vi "two stepper.vi"() -> ()   [LabVIEW 2018]
uses:
  <vilib>/LabVIEW Interface for Arduino/Type Defs/Board Type.ctl
  <vilib>/LabVIEW Interface for Arduino/Type Defs/Connection Type.ctl
  <vilib>/LabVIEW Interface for Arduino/LabVIEW Interface for Arduino.lvlib
panel:
  out "# steps moved":i32
  in  "OK Button":bool
  in  "?":i8(slide) step=2 scale=0.0..2.0
  in  "MOTION":bool
  out "stop motion":bool
  out "Moving?":bool
  in  "Stop":bool
  in  "Arbitray Movement":bool
  in  "# of Steps to Move":i16
  out "Error":errorcluster
  in  "# of translation Steps":i16
  out "Steps Remaining?":bool
  out "Iteration #":i32
  in  "Baud Rate":u32=115200
  out "Step Angle":dbl
  in  "Step Size":i16
  out "Steps Remaining?":bool
  in  "Set Speed (Steps/s)":i16=100 min=0 max=3000 step=50
  in  "Steps for 1 rotation":i16
  in  "Board Type (Uno)":T1
  in  "VISA resource":refnum<visa-resource-name>
  # "For Rotational motion"
  # "For Translational Motion"
  # "OFF"
  # "ON"
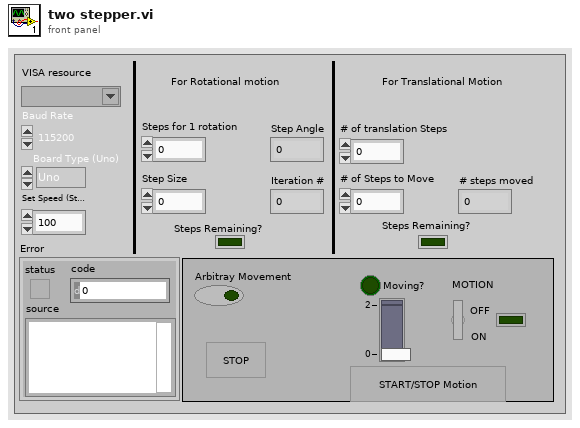
[diagram p1: front panel]
types:
  T1 = typedef "LabVIEW Interface for Arduino.lvlib/Board Type.ctl" = enum16{"Uno", "Dimuelanove w/Atmega 328", "Mega 2560"}
  T2 = typedef "LabVIEW Interface for Arduino.lvlib/Connection Type.ctl" = enum8{"USB / Serial", "XBEE", "BlueSmirf (Bluetooth)"}
  T3 = typedef "LabVIEW Interface for Arduino.lvlib/Arduino Resource.ctl" = cluster{"VISA resource":refnum<visa-resource-name>, "Board Type":T1, "Connection Type":enum8{"USB / Serial"}, "Bytes Per Packet (15)":u8}
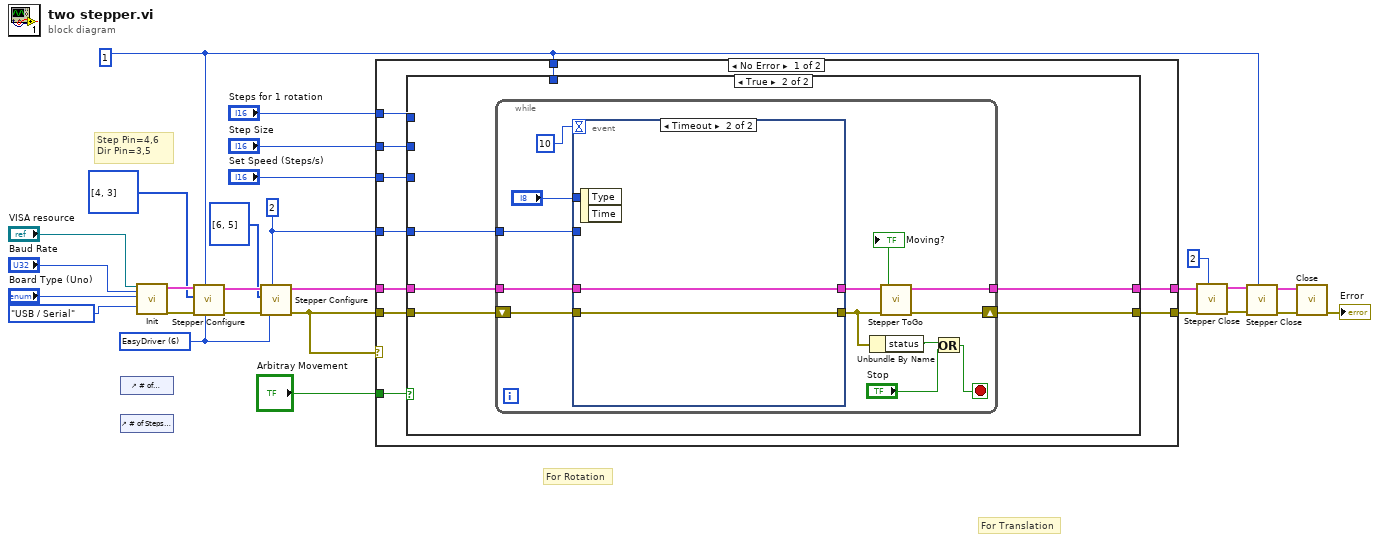
[diagram p0: block diagram]
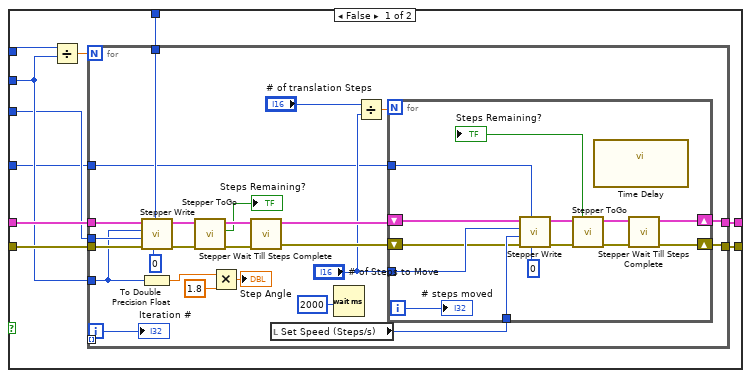
[diagram p2: hidden frame]
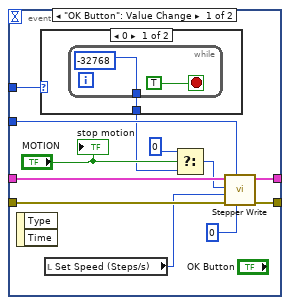
[diagram p3: hidden frame]
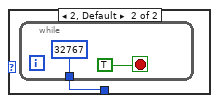
[diagram p4: hidden frame]
diagram:
  w1 = u8 2 ("Stepper #")
  w4 = u8 1 ("Stepper #")
  w2 = u8 6 items=["2 Wire (Pulse & Direction)"=1, "2 Wire"=2, "4 Wire"=4, "EasyDriver"=6, "AF Motor Shield (Stepper 1 & 2 Only)"=5] ("Control Method")
  # "For Translation"
  # "For Rotation"
  # "Step Pin=4,6\nDir Pin=3,5"
  n1 = control-ref of="# of translation Steps"() -> ()  [unwired: 1 out]
  n2 = control-ref of="# of Steps to Move"() -> ()  [unwired: 1 out]
  n3 = call <vilib>:"Init.vi"("VISA resource"="VISA resource", "Baud Rate (115200)"="Baud Rate", "Board Type (Uno)"="Board Type (Uno)", "Connection Type (USB/Serial)"=Connection_Type."USB / Serial") -> ("Arduino Resource"=w24:T3, "error out"=w23:errorcluster)  [unwired: 14 in]
  n4 = call <vilib>:"Stepper Configure.vi"("Control Method"=w2, "Stepper #"=w4, "error in"=w23, "Stepper Pins"=u8[] [4, 3], "Arduino Resource"=w24) -> ("error out"=w6:errorcluster, "Arduino Resource Out"=w8:T3)  [unwired: 5 in]
  n5 = call <vilib>:"Stepper Configure.vi"("Control Method"=w2, "Stepper #"=w1, "error in"=w6, "Stepper Pins"=u8[] [6, 5], "Arduino Resource"=w8) -> ("error out"=w5:errorcluster, "Arduino Resource Out"=w7:T3)  [unwired: 5 in]
  n6 = case shown="No Error" w5 {
    tunnel: [w29 w126] -> w15
    tunnel: [w37 w125] -> w14
    tunnel: w5 -> [w36 w126]
    tunnel: w7 -> [w35 w125]
    tunnel: "Step Size" -> [w34 _]
    tunnel: "Steps for 1 rotation" -> [w33 _]
    tunnel: "Set Speed (Steps/s)" -> [w32 _]
    tunnel: "Arbitray Movement" -> [w31 _]
    tunnel: w4 -> [w30 _]
    tunnel: w1 -> [w28 _]
    frame No Error {
      n7 = case shown="True" w31 {
        tunnel: [w46 w91] -> w37
        tunnel: w36 -> [w45 w88]
        tunnel: w35 -> [w44 w89]
        tunnel: w34 -> [w42 _]
        tunnel: w33 -> [w41 _]
        tunnel: w32 -> [w40 _]
        tunnel: w30 -> [w39 _]
        tunnel: [w47 w90] -> w29
        tunnel: w28 -> [w38 w87]
        frame False {
          n8 = Divide(x=w41, y=w42) -> (x/y=w43:dbl)
          n9 = for {
            N: w43 -> [_]
            tunnel: [w57] -> w47
            tunnel: [w58] -> w46
            tunnel: w45 -> [w69]
            tunnel: w40 -> [w68]
            tunnel: w44 -> [w67]
            tunnel: [w61] -> _ mode=indexing
            tunnel: w42 -> [w60]
            tunnel: w39 -> [w50]
            tunnel: w38 -> [w49]
            i -> [w61]
            n10 = call <vilib>:"Stepper Write.vi"("Set Acceleration (0 to disable)"=i16 0 ("Acceleration"), "Stepper #"=w50, "error in"=w69, "Set Speed (Steps per Second)"=w68, "# of Steps to Move"=w60, "Arduino Resource"=w67) -> ("error out"=w66:errorcluster, "Arduino Resource Out"=w65:T3)  [unwired: 4 in]
            n11 = To Double Precision Float(number=w60) -> (double precision float=w63:dbl)
            n12 = call <vilib>:"Stepper ToGo.vi"("error in"=w66, "Arduino Resource"=w65) -> ("error out"=w72:errorcluster, "Steps Remaining?"=→"Steps Remaining?":bool, "Arduino Resource Out"=w71:T3)  [unwired: 6 in, 1 out]
            n13 = Multiply(x=w63, y=1.8) -> (x*y=→"Step Angle":dbl)
            n14 = call <vilib>:"Stepper Wait Till Steps Complete.vi"("error in"=w72, "Arduino Resource In"=w71) -> ("error out"=w59:errorcluster, "Arduino Resource Out"=w56:T3)  [unwired: 8 in]
            n15 = local read "Set Speed (Steps/s)"() -> (w52:i16)
            n16 = Wait (ms)(milliseconds to wait=u32 2000) -> ()  [unwired: 1 out]
            n17 = Divide(x="# of translation Steps", y="# of Steps to Move") -> (x/y=w55:dbl)
            n18 = for {
              N: w55 -> [_]
              shift-right: [w81] -> w58
              shift-left: w56 -> [w77]
              shift-right: [w80] -> w57
              shift-left: w59 -> [w76]
              tunnel: "# of Steps to Move" -> [w79]
              tunnel: w52 -> [w78]
              tunnel: w49 -> [w73]
              i -> [w74]
              n19 = call <vilib>:"Stepper Write.vi"("Set Acceleration (0 to disable)"=i16 0, "Stepper #"=w73, "error in"=w76, "Set Speed (Steps per Second)"=w78, "# of Steps to Move"=w79, "Arduino Resource"=w77) -> ("error out"=w83:errorcluster, "Arduino Resource Out"=w82:T3)  [unwired: 4 in]
              n20 = call <vilib>:"Stepper ToGo.vi"("error in"=w83, "Arduino Resource"=w82) -> ("error out"=w86:errorcluster, "Steps Remaining?"=→"Steps Remaining?":bool, "Arduino Resource Out"=w85:T3)  [unwired: 6 in, 1 out]
              n21 = call "Time Delay"() -> ()  [unwired: 11 in, 1 out]
              n22 = call <vilib>:"Stepper Wait Till Steps Complete.vi"("error in"=w86, "Arduino Resource In"=w85) -> ("error out"=w80:errorcluster, "Arduino Resource Out"=w81:T3)  [unwired: 8 in]
              "# steps moved" <- w74
            }
            "Iteration #" <- w61
          }
        }
        frame True {
          n23 = while {
            shift-right: [w96] -> w90
            shift-left: w88 -> [w104]
            tunnel: [w95] -> w91
            tunnel: w89 -> [w94]
            tunnel: w87 -> [w93]
            stop <- w102 stop-if-true
            n24 = event shown="[1] Timeout" {
              selector: _ -> [_ _]
              dyn-events: _ -> [_ _]
              timeout: 10 -> [_ _]
              tunnel: w104 -> [w115 w123]
              tunnel: w94 -> [w113 w124]
              tunnel: [w114 w124] -> w100
              tunnel: [w116 w123] -> w98
              tunnel: w93 -> [w109 _]
              tunnel: "?" -> [w107 _]
              event "OK Button": Value Change {
                n25 = event-data() -> ()  [unwired: 1 in, 2 out]
                n26 = case shown="0" w107 {
                  tunnel: [w117 w120] -> w105
                  frame 0 {
                    n27 = while {
                      tunnel: [i16 -32768 ("# of Steps to Move")] -> w117
                      stop <- TRUE ("Stop Reverse movement") stop-if-true
                    }
                  }
                  frame 2, Default {
                    n28 = while {
                      tunnel: [i16 32767 ("# of Steps to Move")] -> w120
                      stop <- TRUE ("Stop Forward movement") stop-if-true
                    }
                  }
                }
                n29 = local read "Set Speed (Steps/s)"() -> (w108:i16)
                n30 = Select(t=0, s="MOTION", f=w105) -> (s? t:f=w110:i32)
                n31 = call <vilib>:"Stepper Write.vi"("Set Acceleration (0 to disable)"=i16 0 ("Set acceleration"), "Stepper #"=w109, "error in"=w115, "Set Speed (Steps per Second)"=w108, "# of Steps to Move"=w110, "Arduino Resource"=w113) -> ("error out"=w116:errorcluster, "Arduino Resource Out"=w114:T3)  [unwired: 4 in]
                "stop motion" <- "MOTION"
              }
              event Timeout {
                n32 = event-data() -> ()  [unwired: 1 in, 2 out]
              }
            }
            n33 = Unbundle By Name(w98) -> ("status"=w101:bool)
            n34 = call <vilib>:"Stepper ToGo.vi"("error in"=w98, "Arduino Resource"=w100) -> ("error out"=w96:errorcluster, "Steps Remaining?"=→"Moving?":bool, "Arduino Resource Out"=w95:T3)  [unwired: 6 in, 1 out]
            n35 = Or(x=w101, y="Stop") -> (x .or. y?=w102:bool)
          }
        }
      }
    }
    frame Error {
    }
  }
  n36 = call <vilib>:"Stepper Close.vi"("Stepper #"=u8 2, "error in"=w15, "Arduino Resource"=w14) -> ("error out"=w16:errorcluster, "Arduino Resource Out"=w17:T3)  [unwired: 7 in]
  n37 = call <vilib>:"Stepper Close.vi"("Stepper #"=w4, "error in"=w16, "Arduino Resource"=w17) -> ("error out"=w20:errorcluster, "Arduino Resource Out"=w21:T3)  [unwired: 7 in]
  n38 = call <vilib>:"Close.vi"("Arduino Resource"=w21, "error in"=w20) -> ("error out"=→"Error":errorcluster)  [unwired: 13 in]
